vi "CloseTcpMessageConnection.vi"(8 "error in (no error)":errorcluster, 11 "connection ID in":T1) -> (0 "error out":errorcluster)   [LabVIEW 2017]
uses:
  <vilib>/addons/InsightCM/MessageBus/TcpApi/controls/TcpMessageReference.ctl
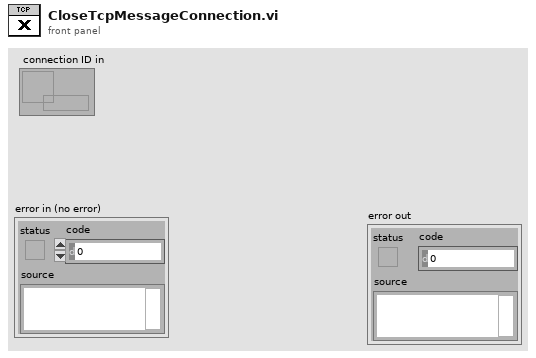
[diagram p1: front panel]
types:
  T1 = typedef "TcpMessageReference.ctl" = refnum<data-value>
  T2 = cluster{"DeviceId":string, "CmdStream":refnum<k5>, "FileStream":refnum<k5>}
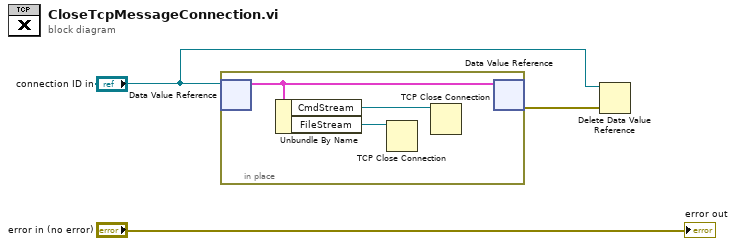
[diagram p0: block diagram]
diagram:
  n1 = in-place {
    n2 = in-place-dvr #1("connection ID in") -> (w4:T2)  [unwired: 1 out]
    n3 = Unbundle By Name(w4) -> ("CmdStream"=w6:refnum<k5>, "FileStream"=w5:refnum<k5>)
    n4 = TCP Close Connection(connection ID=w5) -> ()  [unwired: 2 in, 2 out]
    n5 = TCP Close Connection(connection ID=w6) -> ()  [unwired: 2 in, 2 out]
    n6 = in-place-dvr #1(w4) -> (w2:errorcluster)  [unwired: 1 out]
  }
  n7 = Delete Data Value Reference(data value reference="connection ID in", error in=w2) -> ()  [unwired: 2 out]
  "error out" <- "error in (no error)"
